vi "CalcCoilsBytes.vi"(10 "Value":u16) -> (2 "数值":u32)   [LabVIEW 2015]
doc: "根据线圈数量计算占用多少个字节（8Bits）\n输出占用的的字节数量"
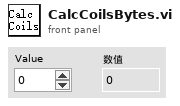
[diagram p1: front panel]
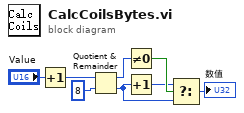
[diagram p0: block diagram]
diagram:
  n1 = Increment(x="Value") -> (x+1=w1:u16)
  n2 = Quotient & Remainder(x=w1, y=u32 8) -> (x-y*floor(x/y)=w6:u32, floor(x/y)=w7:u32)
  n3 = Not Equal To 0?(x=w6) -> (x != 0?=w5:bool)
  n4 = Increment(x=w7) -> (x+1=w4:u32)
  n5 = Select(t=w4, s=w5, f=w7) -> (s? t:f=→"数值":u32)
